vi "load_avi_to_stack.vi"(8 "Image Prefix":string="raw", 9 "Preview":bool, 10 "AVI File":path=path "\\\\healey\\aog/general storage/REBOT/B Scan Assembly/Dataset 1 Scanner/data/j9b.avi", 11 "Preview IMAQ":T1) -> (2 "Image Array":T1[](array[typedef]), 3 "Num Images":i32=1)   [LabVIEW 2016]
doc: "Loads an AVI to a stack of IMAQ images."
uses:
  <vilib>/vision/Image Controls.llb/IMAQ Image.ctl
panel:
  out "error out":errorcluster
  in  "error in (no error)":errorcluster
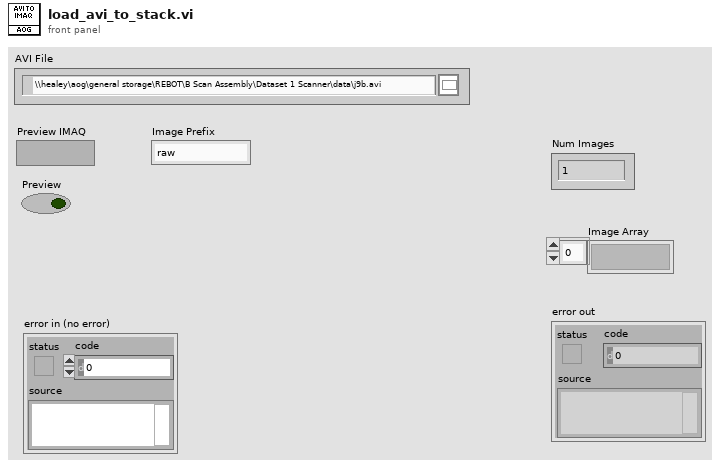
[diagram p1: front panel]
types:
  T1 = typedef "IMAQ Image.ctl" = refnum<image>
  T2 = typedef "Image Type" = u32
  T3 = typedef "IMAQ AVI2 Refnum.ctl" = refnum<k20>
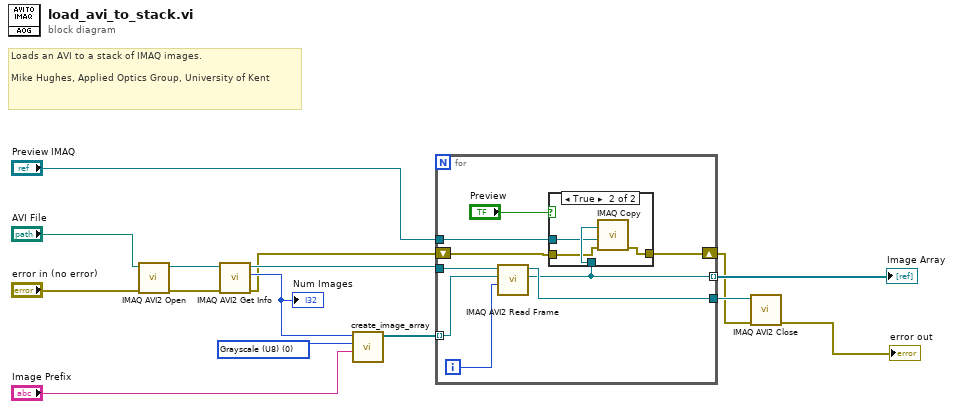
[diagram p0: block diagram]
diagram:
  w7 = T2 0 items=["Grayscale (U8)", "Grayscale (I16)", "Grayscale (SGL)", "Complex (CSG)", "RGB (U32)", "HSL (U32)", "RGB (U64)", "Grayscale (U16)"] ("Image Type")
  # "Loads an AVI to a stack of IMAQ images.\n\nMike Hughes, Applied Optics Group, University of Kent"
  n1 = call "IMAQ AVI2 Open"("error in (no error)"="error in (no error)", "AVI File Path"="AVI File") -> ("error out"=w4:errorcluster, "AVI Refnum"=w6:T3)  [unwired: 8 in]
  n2 = call "IMAQ AVI2 Get Info"("error in (no error)"=w4, "AVI Refnum"=w6) -> ("error out"=w3:errorcluster, "Number of Frames"=w14:u32, "AVI Refnum (duplicate)"=w8:T3)  [unwired: 5 in, 2 out]
  "Num Images" <- w14
  n3 = call "create_image_array.vi"("Prefix"="Image Prefix", "Image Type"=w7, "Num Images"=w14) -> ("Image Array"=w12:T1[])  [unwired: 7 in, 1 out]
  n4 = for {
    tunnel: w12 -> [w23] mode=indexing
    tunnel: w8 -> [w24]
    tunnel: [w22] -> w10
    tunnel: [w20] -> w13 mode=indexing
    tunnel: "Preview IMAQ" -> [w19]
    shift-right: [w16] -> w2
    shift-left: w3 -> [w17]
    i -> [w21]
    n5 = call "IMAQ AVI2 Read Frame"("Frame Number"=w21, "Image"=w23, "AVI Refnum"=w24) -> ("Image Out"=w20:T1, "AVI Refnum (duplicate)"=w22:T3)  [unwired: 6 in, 1 out]
    n6 = case shown="True" "Preview" {
      tunnel: w20 -> [_ w29]
      tunnel: w19 -> [_ w28]
      tunnel: w17 -> [w25 w27]
      tunnel: [w25 w26] -> w16
      frame False {
      }
      frame True {
        n7 = call "IMAQ Copy"("error in (no error)"=w27, "Image Dst"=w28, "Image Src"=w29) -> ("error out"=w26:errorcluster)  [unwired: 3 in, 1 out]
      }
    }
  }
  "Image Array" <- w13
  n8 = call "IMAQ AVI2 Close"("error in (no error)"=w2, "AVI Refnum"=w10) -> ("error out"=→"error out":errorcluster)  [unwired: 9 in]
